vi "check for recovery.vi"(8 "error in (no error)":errorcluster, 9 "run flags in":u8, 10 "error in":errorcluster, 11 "TBM module execution interface in":refnum<class "TBM module execution interface.lvclass">) -> (0 "error out":errorcluster, 1 "run flags out":u8, 2 "error":errorcluster, 3 "TBM module execution interface out":refnum<class "TBM module execution interface.lvclass">)   [LabVIEW 2013]
uses:
  <vilib>/NI/Tag Bus Module Framework/runtime/TBM module execution interface.lvclass
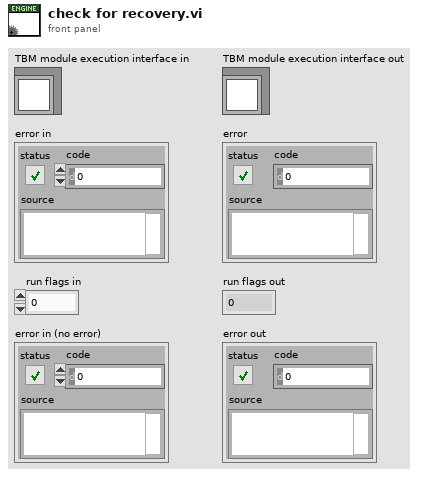
[diagram p1: front panel]
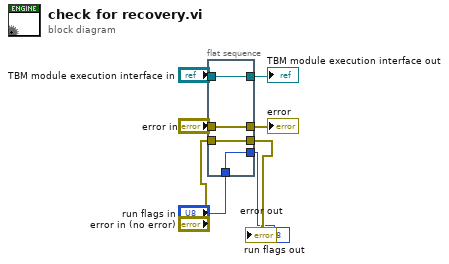
[diagram p0: block diagram]
diagram:
  n1 = flat-sequence {
    tunnel: [w12] -> w1
    tunnel: "TBM module execution interface in" -> [w12]
    tunnel: "error in" -> [w11]
    tunnel: [w11] -> w4
    tunnel: [w10] -> w5
    tunnel: "run flags in" -> [w10]
    tunnel: "error in (no error)" -> [w9]
    tunnel: [w9] -> w8
    frame #0 {
    }
  }
  "error out" <- w8
  "run flags out" <- w5
  "error" <- w4
  "TBM module execution interface out" <- w1
